vi "DHE_samplingsfromDBS.vi"(8 "error in (no error)":errorcluster, 11 "Database RefNum in":T1) -> (0 "error out":errorcluster, 1 "coadds":i32, 2 "fsamples":i32, 3 "exptime":i32, 4 "nimages":i32, 5 "readtime":sgl, 6 "sur":i32)   [LabVIEW 2016]
uses:
  DBSHAND/private/vis/DatabaseHand_RefNum.ctl
  DBSHAND/private/vis/DatabaseHand_Element_Get(double).vi
  DBSHAND/private/vis/DatabaseHand_Element_Get(I32).vi
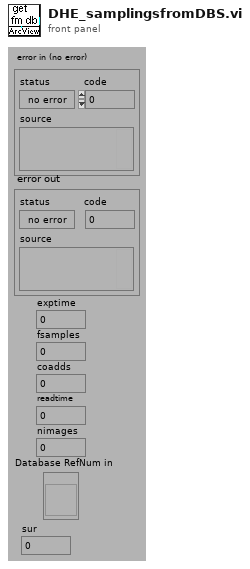
[diagram p1: front panel]
types:
  T1 = typedef "DatabaseHand_RefNum.ctl" = refnum<vi>
  T2 = typedef "CMN_ContStatus.ctl" = cluster{"Response":string, "power":bool, "shutter":bool, "artifdata":bool, "idlemode":bool, "reset":bool, "gain":i32, "speed":i32, "resetPCI":bool, "autoshutter":bool, "TempSetPoint":i32, "multipleextensions":bool, "displayImage":bool, "coadding":bool, "images being coadded":i32, "Operation Mode":enum16{"normal", "coadd", "fawler"}, "frames to write":cluster{"subs":bool, "reset":bool, "exposed":bool}, "fawler samples":i32, "write auto":bool, "datatype":string, "frames to display":cluster{"subs":bool, "reset":bool, "exposed":bool}, "sur":i32, "autoclear":bool}
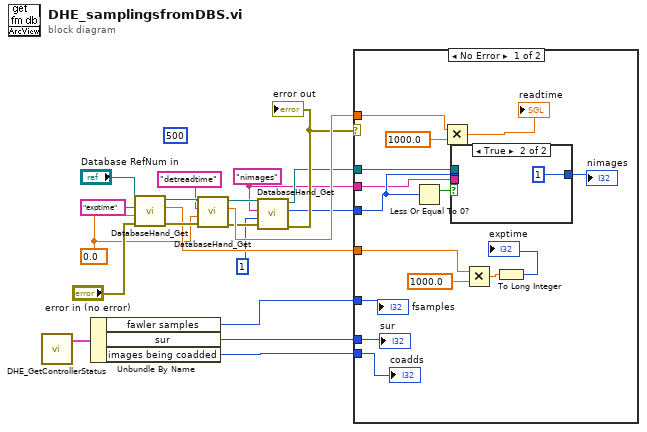
[diagram p0: block diagram]
diagram:
  w1 = "nimages" ("name")
  w12 = 0.0
  (unwired) 500 ("ms timeout (-1)")
  n1 = call "DHE_GetControllerStatus.vi"() -> ("ControllerStatus"=w20:T2)  [unwired: 11 out]
  n2 = Unbundle By Name(w20) -> ("fawler samples"=w5:i32, "sur"=w4:i32, "images being coadded"=w3:i32)
  n3 = call-poly "DatabaseHand_Get.vi"("error in (no error)"="error in (no error)", "default value"=w12, "name"="exptime", "Database RefNum in"="Database RefNum in") -> ("error out"=w14:errorcluster, "value"=w13:dbl, "Database RefNum out"=w17:T1)  [unwired: 1 in, 4 out]
  n4 = call-poly "DatabaseHand_Get.vi"("error in (no error)"=w14, "default value"=w12, "name"="detreadtime", "Database RefNum in"=w17) -> ("error out"=w10:errorcluster, "value"=w11:dbl, "Database RefNum out"=w9:T1)  [unwired: 1 in, 4 out]
  n5 = call-poly "DatabaseHand_Get.vi"("error in (no error)"=w10, "default value"=1, "name"=w1, "Database RefNum in"=w9) -> ("error out"=w7:errorcluster, "value"=w6:i32, "Database RefNum out"=w2:T1)  [unwired: 1 in, 4 out]
  "error out" <- w7
  n6 = case shown="No Error" w7 {
    tunnel: w13 -> [w31 _]
    tunnel: w11 -> [w30 _]
    tunnel: w6 -> [w25 _]
    tunnel: w5 -> [w29 _]
    tunnel: w4 -> [w28 _]
    tunnel: w3 -> [w27 _]
    tunnel: w2 -> [w23 _]
    tunnel: w1 -> [w22 _]
    frame No Error {
      n7 = Less Or Equal To 0?(x=w25) -> (x <= 0?=w26:bool)
      n8 = Multiply(x=w30, y=1000.0) -> (x*y=→"readtime":dbl)
      n9 = case shown="True" w26 {
        tunnel: w25 -> [w36 _]
        tunnel: [w36 1 ("value")] -> w24
        tunnel: w23 -> [_ _]
        tunnel: w22 -> [_ _]
        frame False {
        }
        frame True {
        }
      }
      "nimages" <- w24
      n10 = Multiply(x=w31, y=1000.0) -> (x*y=w34:dbl)
      n11 = To Long Integer(number=w34) -> (32bit integer=→"exptime":i32)
      "fsamples" <- w29
      "sur" <- w28
      "coadds" <- w27
    }
    frame Error {
    }
  }
